vi "Test App Removed App Nested Process Context Removed.vi"(8 "error in (no error)":errorcluster, 11 "Rig Test in":refnum<class "Application Test.lvclass">) -> (0 "error out":errorcluster, 3 "Rig Test out":refnum<class "Application Test.lvclass">)   [LabVIEW 2020, in "Application Test.lvclass"]
uses:
  Application Test.lvclass
  C:/Program Files (x86)/National Instruments/LabVIEW 2020/vi.lib/Asteme/LUnit/Test Case.lvclass
  Framework/Process/Process.lvclass
  Framework/Application/Application.lvclass
  C:/Users/anton/Documents/GitHub/Triarc-Framework/source/Framework/Process/Process.lvclass
  Framework/Process/Process.lvclass/Process.ctl
  Framework/Application/Application.lvclass/Application.ctl
  <vilib>/Asteme/LUnit/Test Case.lvclass/Test Case.ctl
  <vilib>/Asteme/LUnit/LUnit Assertion Result.lvclass/LUnit Assertion Result.ctl
  Framework/Application/Private/Add Process to Map.vi
  Framework/Application/Private/Start Idle Processes if Running.vi
  Framework/Process/Protected/Messaging/Enqueue Message.vi
  Framework/Process/Public/Lifecycle/Get Lifecycle State.vi
  Framework/Process/Protected/SubVIs/Set Context.vi
  <vilib>/Asteme/LUnit/Palette/Pass.vi
  <vilib>/Asteme/LUnit/Palette/Fail.vi
  <vilib>/Asteme/LUnit/Variant to string.vi
  <vilib>/Asteme/LUnit/Set Assertion Type.vi
  Framework/Process/Private/SubVIs/Wait for finish.vi
  Framework/Process/Private/SubVIs/Set Lifecycle State.vi
  <vilib>/Utility/error.llb/Clear Errors.vi
  Framework/Process/Public/Lifecycle/Leave Process Loop.vi
  <vilib>/Asteme/LUnit/Add test result.vi
  <vilib>/Asteme/LUnit/LUnit Write Passed.vi
  <vilib>/Asteme/LUnit/LUnit Get Test Case.vi
  <vilib>/Asteme/LUnit/Assertion Result/LUnit Get Test Name.vi
  <vilib>/Asteme/LUnit/LUnit Write Message.vi
  <vilib>/Asteme/LUnit/LUnit Write Description.vi
  <vilib>/Asteme/LUnit/LUnit Write Assertion Type.vi
  <vilib>/Asteme/LUnit/Read Test Case Name.vi
  <vilib>/Utility/error.llb/Error Cluster From Error Code.vi
  Framework/Application/Private/Throw Error If Process Already in App.vi
  Framework/Application/Private/Update Context for Owned Processes.vi
  <vilib>/Utility/Data Type/Get Type Information.vi
  <vilib>/Utility/LVClass/Get LV Class Name.vi
  <vilib>/Asteme/LUnit/LUnit Assertion Result.lvclass
  <vilib>/Asteme/LUnit/Test Case.lvclass
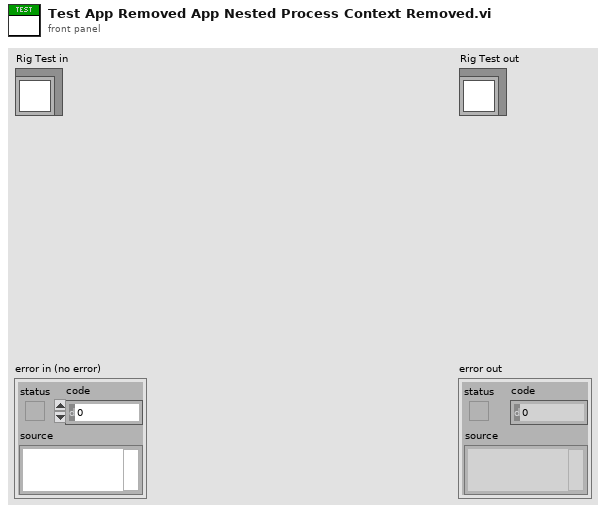
[diagram p1: front panel]
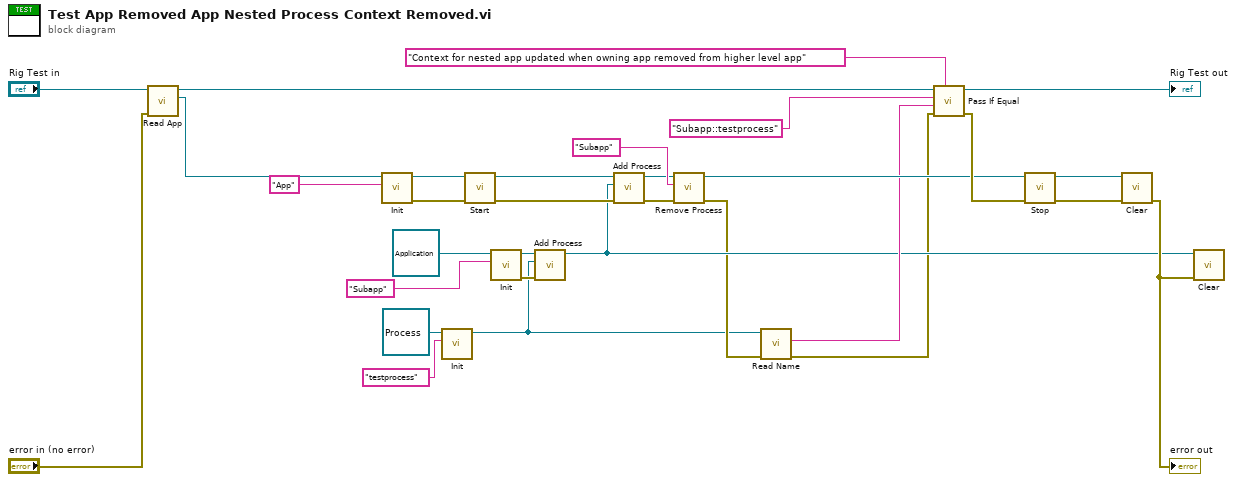
[diagram p0: block diagram]
diagram:
  n1 = call "Read App.vi"("error in (no error)"="error in (no error)", "Application Test In"="Rig Test in") -> ("App out"=w30:refnum<class "Application.lvclass">, "Application Test Out"=w20:refnum<class "Application Test.lvclass">)  [unwired: 7 in, 1 out]
  n2 = call-dynamic "Init.vi"("Name"="App", "Process In"=w30) -> ("error out"=w21:errorcluster, "Process Out"=w22:refnum<class "Application.lvclass">)  [unwired: 8 in]
  n3 = call-dynamic "Init.vi"("Name"="testprocess", "Process In"=refnum<class "Process.lvclass"> refnum ("Process.lvclass")) -> ("Process Out"=w3:refnum<class "Process.lvclass">)  [unwired: 8 in, 1 out]
  n4 = call "Start.vi"("error in (no error)"=w21, "Process In"=w22) -> ("error out"=w23:errorcluster, "Process Out"=w15:refnum<class "Application.lvclass">)  [unwired: 7 in, 1 out]
  n5 = call-dynamic "Init.vi"("Name"="Subapp", "Process In"=refnum<class "Application.lvclass"> refnum ("App out")) -> ("error out"=w8:errorcluster, "Process Out"=w9:refnum<class "Application.lvclass">)  [unwired: 8 in]
  n6 = call "Add Process.vi"("error in (no error)"=w8, "Process"=w3, "Rig In"=w9) -> ("Rig Out"=w6:refnum<class "Application.lvclass">)  [unwired: 7 in, 1 out]
  n7 = call "Add Process.vi"("error in (no error)"=w23, "Process"=w6, "Rig In"=w15) -> ("error out"=w27:errorcluster, "Rig Out"=w1:refnum<class "Application.lvclass">)  [unwired: 7 in]
  n8 = call "Remove Process.vi"("error in (no error)"=w27, "Process Name"="Subapp" ("Name"), "Rig In"=w1) -> ("error out"=w5:errorcluster, "Rig Out"=w16:refnum<class "Application.lvclass">)  [unwired: 6 in, 1 out]
  n9 = call "Read Name.vi"("error in (no error)"=w5, "Process In"=w3) -> ("error out"=w4:errorcluster, "Qualified Name"=w12:string)  [unwired: 6 in, 2 out]
  n10 = call <vilib>:"Pass If Equal.vi"("Description"="Context for nested app updated when owning app removed from higher level app", "error in (no error)"=w4, "Actual"=w12, "Expected"="Subapp::testprocess" ("Name"), "Test Case In"=w20) -> ("error out"=w25:errorcluster, "Test Case Out"=→"Rig Test out":refnum<class "Application Test.lvclass">)  [unwired: 5 in]
  n11 = call "Stop.vi"("error in (no error)"=w25, "Process In"=w16) -> ("error out"=w18:errorcluster, "Process Out"=w17:refnum<class "Application.lvclass">)  [unwired: 7 in, 1 out]
  n12 = call-dynamic "Clear.vi"("error in (no error)"=w18, "Application In"=w17) -> ("error out"=w14:errorcluster)  [unwired: 9 in]
  "error out" <- w14
  n13 = call-dynamic "Clear.vi"("error in (no error)"=w14, "Application In"=w6) -> ()  [unwired: 9 in, 1 out]
